vi "GetXMLValueForTag.vi"(8 "error in (no error)":errorcluster, 9 "tag":string, 11 "XML":string) -> (0 "error out":errorcluster, 3 "value":string)   [LabVIEW 2009, in "NavScreen.lvlib"]
uses:
  NavScreen.lvlib
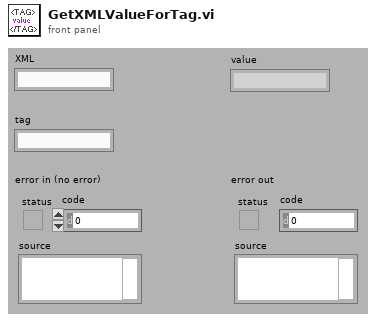
[diagram p1: front panel]
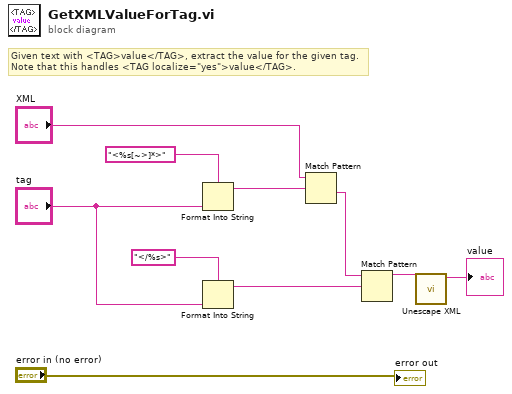
[diagram p0: block diagram]
diagram:
  # "Given text with <TAG>value</TAG>, extract the value for the given tag.\nNote that this handles <TAG localize=\"yes\">value</TAG>."
  n1 = Format Into String(format string="<%s[~>]*>" ("regular expression"), "tag") -> (resulting string=w5:string)  [unwired: 2 in, 1 out]
  n2 = Format Into String(format string="</%s>" ("regular expression"), "tag") -> (resulting string=w4:string)  [unwired: 2 in, 1 out]
  n3 = Match Pattern(string="XML", regular expression=w5) -> (after substring=w10:string)  [unwired: 1 in, 3 out]
  n4 = Match Pattern(string=w10, regular expression=w4) -> (before substring=w2:string)  [unwired: 1 in, 3 out]
  n5 = call <vilib>:"Unescape XML.vi"("XML String In"=w2) -> ("XML String Out"=→"value":string)  [unwired: 9 in, 1 out]
  "error out" <- "error in (no error)"
